vi "ProgG_005_kz_MG.vi"(1 "x2":ext=19.4, 2 "x1":ext=14.1) -> (0 "y":dbl=14.105)   [LabVIEW 2021]
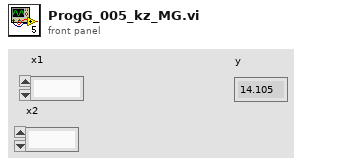
[diagram p1: front panel]
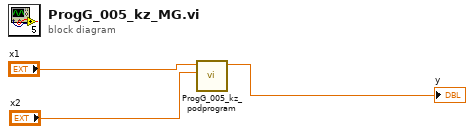
[diagram p0: block diagram]
diagram:
  n1 = call "ProgG_005_kz_podprogram.vi"("x2"="x2", "x1"="x1") -> ("Numeric"=→"y":ext)  [unwired: 9 in]
